vi "All Channel Names.vi"(0 "Data":T2={"AO config"=[], "AI config"=[], "DI config"=[], "DO config"=[], "TC config"=[{"Channel_Name"="", "Channel_Number"="", "Pre_Scale_min"=0.0, "Pre_Scale_max"=0.0, "units"=4, " type"=7}], "ACC config"=[], "SG config"=[], "Strain Gauge Settings"={"poisson ratio"=0.3, "nominal gage resistance"=120.0, "gage factor"=2.08}, "bridge information"={"strain configuration"=10271, "lead wire resistance"=1.7, "initial bridge voltage"=0.0, "voltage excitation source"=10200, "voltage excitation value"=3.3}, "Sample Rate"={"AI Sample Rate"=0.0, "AO Sample Rate"=0.0, "DI Sample Rate"=0.0, "TC Sample Rate"=0.0, "DO Sample Rate"=0.0, "SG Sample Rate"=0.0, "ACC Sample Rate"=0.0}} {"bridge information"."initial bridge voltage" format="%0.2f"; "bridge information"."voltage excitation source" items=["Internal"=10200, "External"=10167, "None"=10230]; "bridge information"."voltage excitation value" format="%0.2f"; "bridge information"."lead wire resistance" format="%0.2f"; "bridge information"."strain configuration" items=["Full Bridge I"=10183, "Full Bridge II"=10184, "Full Bridge III"=10185, "Half Bridge I"=10188, "Half Bridge II"=10189, "Quarter Bridge I"=10271, "Quarter Bridge II"=10272]; "ACC config"."Terminal configuration" items=["default"=-1, "RSE"=10083, "NRSE"=10078, "Differential"=10106, "Pseudodifferential"=12529]; "ACC config"."Sensitivity units" items=["mVolts/g"=12509, "Volts/g"=12510]; "TC config"."type" items=["J"=10072, "K"=10073, "N"=10077, "R"=10082, "S"=10085, "T"=10086, "B"=10047, "E"=10055]; "TC config"."units" items=["Deg C", "Deg F", "Kelvins", "Deg R", "From Custom Scale"]}, 1 "Enum":enum16{"Read", "Write"}(ring)) -> (4 "Channel names":T1, 6 "AO,AI,DI,DO,TC,ACC,SG":i32[](array[numeric]))   [LabVIEW 2022 SP3]
uses:
  Controls/Config.ctl
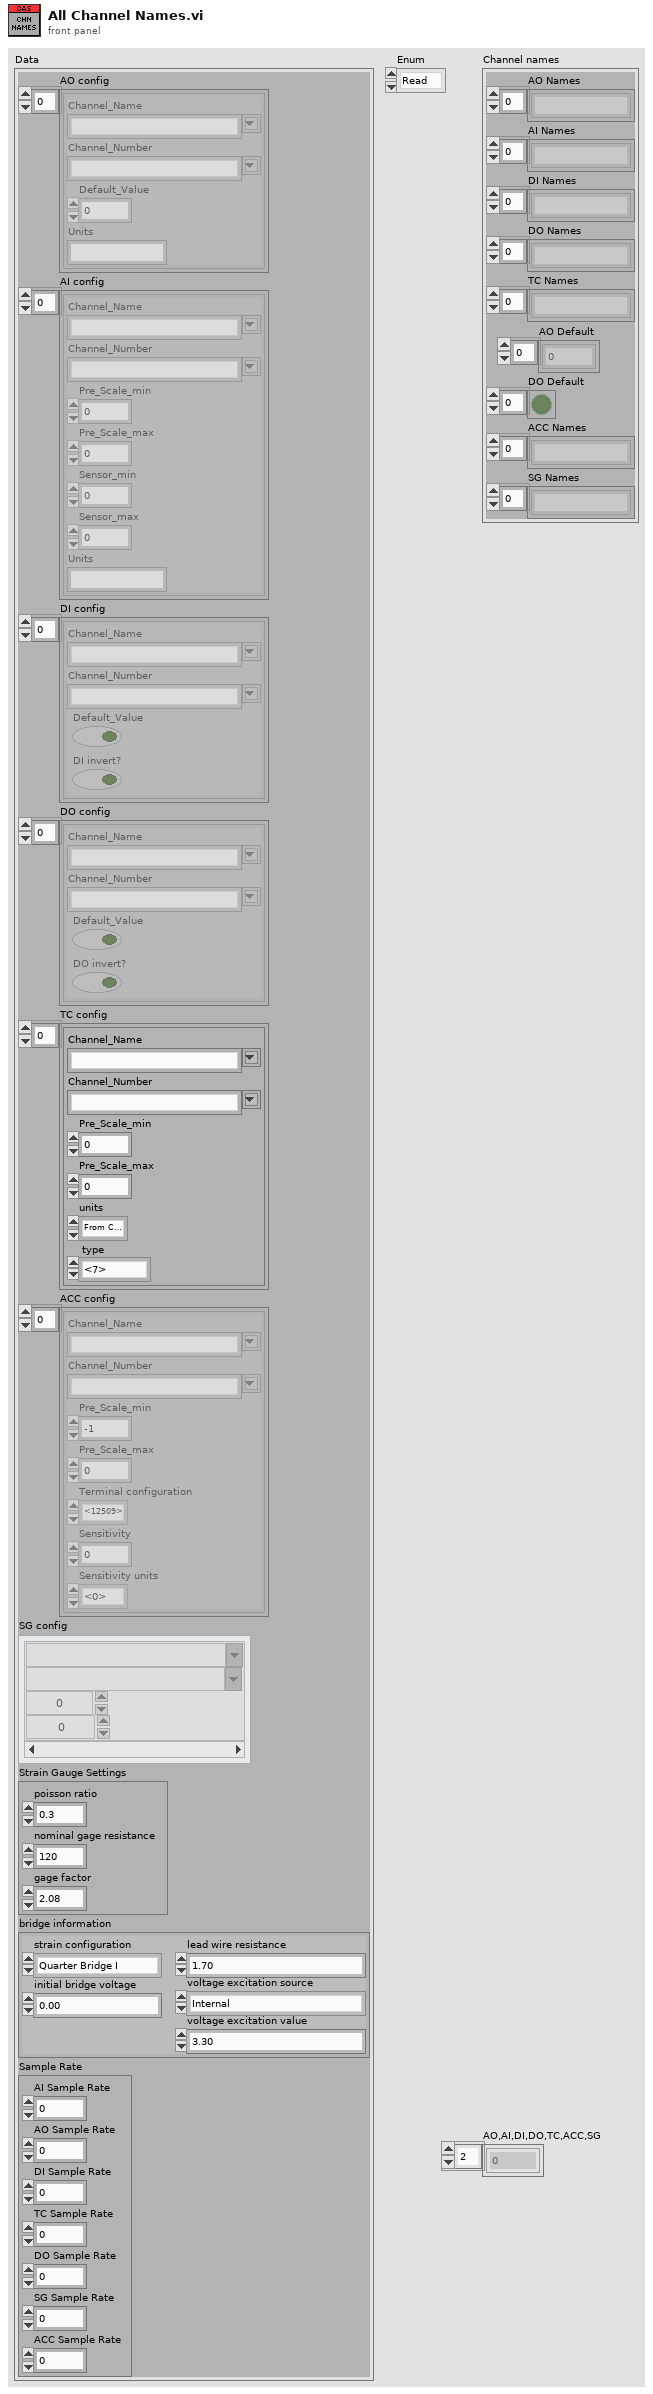
[diagram p1: front panel]
types:
  T1 = cluster{"AO Names":string[], "AI Names":string[], "DI Names":string[], "DO Names":string[], "TC Names":string[], "AO Default":dbl[], "DO Default":bool[], "ACC Names":string[], "SG Names":string[]}
  T2 = typedef "Config.ctl" = cluster{"AO config":cluster{"Channel_Name":string, "Channel_Number":string, "Default_Value":dbl, "Units":string}[], "AI config":cluster{"Channel_Name":string, "Channel_Number":string, "Pre_Scale_min":dbl, "Pre_Scale_max":dbl, "Sensor_min":dbl, "Sensor_max":dbl, "Units":string}[], "DI config":cluster{"Channel_Name":string, "Channel_Number":string, "Default_Value":bool, "DI invert?":bool}[], "DO config":cluster{"Channel_Name":string, "Channel_Number":string, "Default_Value":bool, "DO invert?":bool}[], "TC config":cluster{"Channel_Name":string, "Channel_Number":string, "Pre_Scale_min":dbl, "Pre_Scale_max":dbl, "units":i32, " type":i32}[], "ACC config":cluster{"Channel_Name":string, "Channel_Number":string, "Pre_Scale_min":dbl, "Pre_Scale_max":dbl, "Terminal configuration":i32, "Sensitivity":dbl, "Sensitivity units":i32}[], "SG config":cluster{"Channel_Name":string, "Channel_Number":string, "Pre_Scale_min":dbl, "Pre_Scale_max":dbl}[], "Strain Gauge Settings":cluster{"poisson ratio":dbl, "nominal gage resistance":dbl, "gage factor":dbl}, "bridge information":cluster{"strain configuration":i32, "lead wire resistance":dbl, "initial bridge voltage":dbl, "voltage excitation source":i32, "voltage excitation value":dbl}, "Sample Rate":cluster{"AI Sample Rate":dbl, "AO Sample Rate":dbl, "DI Sample Rate":dbl, "TC Sample Rate":dbl, "DO Sample Rate":dbl, "SG Sample Rate":dbl, "ACC Sample Rate":dbl}}
  T3 = cluster{"Channel_Name":string, "Channel_Number":string, "Default_Value":dbl, "Units":string}[]
  T4 = cluster{"Channel_Name":string, "Channel_Number":string, "Pre_Scale_min":dbl, "Pre_Scale_max":dbl, "Sensor_min":dbl, "Sensor_max":dbl, "Units":string}[]
  T5 = cluster{"Channel_Name":string, "Channel_Number":string, "Default_Value":bool, "DI invert?":bool}[]
  T6 = cluster{"Channel_Name":string, "Channel_Number":string, "Default_Value":bool, "DO invert?":bool}[]
  T7 = cluster{"Channel_Name":string, "Channel_Number":string, "Pre_Scale_min":dbl, "Pre_Scale_max":dbl, "units":i32, " type":i32}[]
  T8 = cluster{"Channel_Name":string, "Channel_Number":string, "Pre_Scale_min":dbl, "Pre_Scale_max":dbl, "Terminal configuration":i32, "Sensitivity":dbl, "Sensitivity units":i32}[]
  T9 = cluster{"Channel_Name":string, "Channel_Number":string, "Pre_Scale_min":dbl, "Pre_Scale_max":dbl}[]
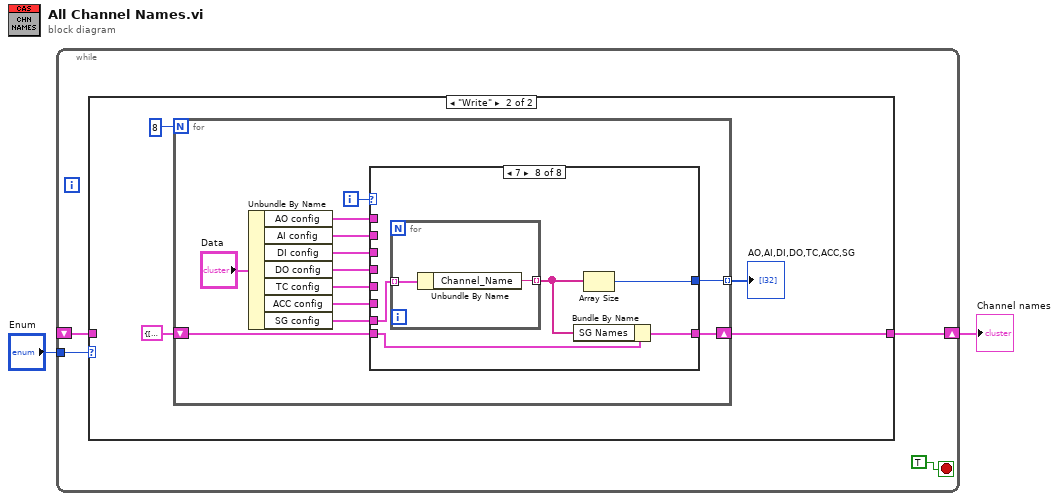
[diagram p0: block diagram]
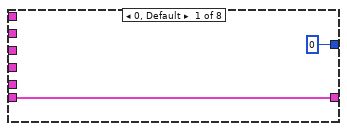
[diagram p3: hidden frame]
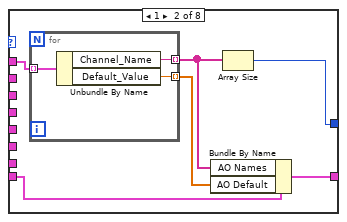
[diagram p4: hidden frame]
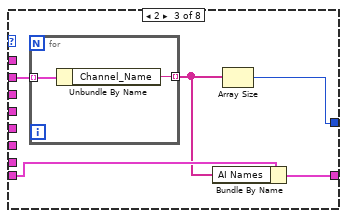
[diagram p5: hidden frame]
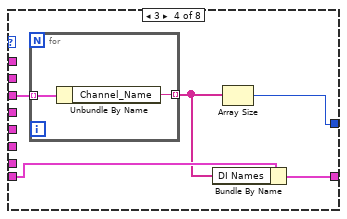
[diagram p6: hidden frame]
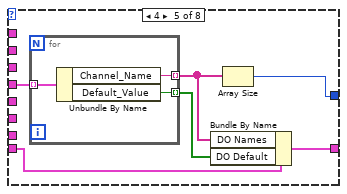
[diagram p7: hidden frame]
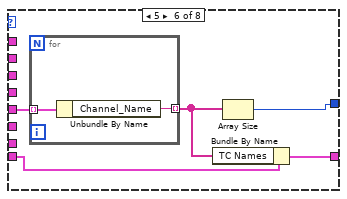
[diagram p8: hidden frame]
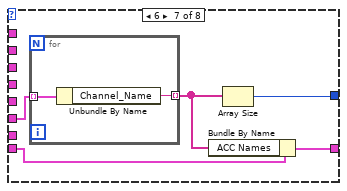
[diagram p9: hidden frame]
diagram:
  n1 = while {
    shift-right: [w5] -> w1
    shift-left: _ -> [w4]
    tunnel: "Enum" -> [w3]
    stop <- TRUE stop-if-true
    n2 = case shown="\"Write\"" w3 {
      tunnel: [w7 w9] -> w5
      tunnel: w4 -> [w7 _]
      frame "Read", Default {
      }
      frame "Write" {
        n3 = for {
          N: 8 -> [_]
          shift-right: [w15] -> w9
          shift-left: T1 {"AO Names"=[], "AI Names"=[], "DI Names"=[], "DO Names"=[], "TC Names"=[], "AO Default"=[], "DO Default"=[], "ACC Names"=[], "SG Names"=[]} ("Chaneel names") -> [w16]
          tunnel: [w12] -> w8 mode=indexing
          i -> [w22]
          n4 = Unbundle By Name("Data") -> ("AO config"=w21:T3, "AI config"=w20:T4, "DI config"=w18:T5, "DO config"=w19:T6, "TC config"=w17:T7, "ACC config"=w14:T8, "SG config"=w13:T9)
          n5 = case shown="7" w22 {
            tunnel: w21 -> [_ w31 _ _ _ _ _ _]
            tunnel: w20 -> [_ _ w39 _ _ _ _ _]
            tunnel: w19 -> [_ _ _ _ w54 _ _ _]
            tunnel: w18 -> [_ _ _ w46 _ _ _ _]
            tunnel: w17 -> [_ _ _ _ _ w62 _ _]
            tunnel: w16 -> [w25 w30 w38 w44 w53 w60 w68 w75]
            tunnel: [w25 w29 w37 w45 w52 w61 w69 w76] -> w15
            tunnel: w14 -> [_ _ _ _ _ _ w67 _]
            tunnel: w13 -> [_ _ _ _ _ _ _ w74]
            tunnel: [0 w26 w36 w42 w49 w59 w66 w73] -> w12
            frame 0, Default {
            }
            frame 1 {
              n6 = for {
                tunnel: w31 -> [w34] mode=indexing
                tunnel: [w33] -> w27 mode=indexing
                tunnel: [w32] -> w28 mode=indexing
                n7 = Unbundle By Name(w34) -> ("Channel_Name"=w33:string, "Default_Value"=w32:dbl)
              }
              n8 = Bundle By Name(cluster=w30, "AO Names"=w27, "AO Default"=w28) -> (w29:T1)
              n9 = Array Size(array=w27) -> (size(s)=w26:i32)
            }
            frame 2 {
              n10 = for {
                tunnel: w39 -> [w41] mode=indexing
                tunnel: [w40] -> w35 mode=indexing
                n11 = Unbundle By Name(w41) -> ("Channel_Name"=w40:string)
              }
              n12 = Bundle By Name(cluster=w38, "AI Names"=w35) -> (w37:T1)
              n13 = Array Size(array=w35) -> (size(s)=w36:i32)
            }
            frame 3 {
              n14 = for {
                tunnel: [w48] -> w43 mode=indexing
                tunnel: w46 -> [w47] mode=indexing
                n15 = Unbundle By Name(w47) -> ("Channel_Name"=w48:string)
              }
              n16 = Bundle By Name(cluster=w44, "DI Names"=w43) -> (w45:T1)
              n17 = Array Size(array=w43) -> (size(s)=w42:i32)
            }
            frame 4 {
              n18 = for {
                tunnel: [w57] -> w50 mode=indexing
                tunnel: w54 -> [w56] mode=indexing
                tunnel: [w55] -> w51 mode=indexing
                n19 = Unbundle By Name(w56) -> ("Channel_Name"=w57:string, "Default_Value"=w55:bool)
              }
              n20 = Bundle By Name(cluster=w53, "DO Names"=w50, "DO Default"=w51) -> (w52:T1)
              n21 = Array Size(array=w50) -> (size(s)=w49:i32)
            }
            frame 5 {
              n22 = for {
                tunnel: [w64] -> w58 mode=indexing
                tunnel: w62 -> [w63] mode=indexing
                n23 = Unbundle By Name(w63) -> ("Channel_Name"=w64:string)
              }
              n24 = Bundle By Name(cluster=w60, "TC Names"=w58) -> (w61:T1)
              n25 = Array Size(array=w58) -> (size(s)=w59:i32)
            }
            frame 6 {
              n26 = for {
                tunnel: [w71] -> w65 mode=indexing
                tunnel: w67 -> [w70] mode=indexing
                n27 = Unbundle By Name(w70) -> ("Channel_Name"=w71:string)
              }
              n28 = Bundle By Name(cluster=w68, "ACC Names"=w65) -> (w69:T1)
              n29 = Array Size(array=w65) -> (size(s)=w66:i32)
            }
            frame 7 {
              n30 = for {
                tunnel: [w78] -> w72 mode=indexing
                tunnel: w74 -> [w77] mode=indexing
                n31 = Unbundle By Name(w77) -> ("Channel_Name"=w78:string)
              }
              n32 = Bundle By Name(cluster=w75, "SG Names"=w72) -> (w76:T1)
              n33 = Array Size(array=w72) -> (size(s)=w73:i32)
            }
          }
        }
        "AO,AI,DI,DO,TC,ACC,SG" <- w8
      }
    }
  }
  "Channel names" <- w1
